vi "Divide.vi"(0 "A":dbl, 5 "B":dbl) -> (4 "C":dbl)   [LabVIEW 2020]
doc: "This vi is a part of polymophic vi which can do division"
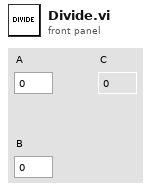
[diagram p1: front panel]
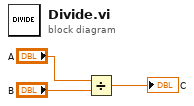
[diagram p0: block diagram]
diagram:
  n1 = Divide(x="A", y="B") -> (x/y=→"C":dbl)
